vi "Test Y Position Data.vi"() -> (0 "Reason":string, 1 "Success":bool)   [LabVIEW 2013]
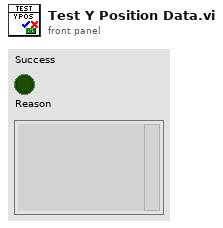
[diagram p1: front panel]
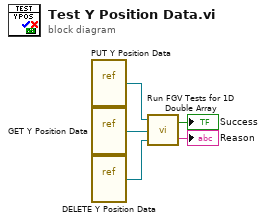
[diagram p0: block diagram]
diagram:
  n1 = vi-ref "PUT Y Position Data.vi"() -> (w4:refnum<vi>)
  n2 = vi-ref "GET Y Position Data.vi"() -> (w5:refnum<vi>)
  n3 = vi-ref "DELETE Y Position Data.vi"() -> (w3:refnum<vi>)
  n4 = call "Run FGV Tests for 1D Double Array.vi"("DELETE VI Reference"=w3, "GET VI Reference"=w5, "PUT VI Reference"=w4) -> ("Reason"=→"Reason":string, "Success"=→"Success":bool)
